vi "Actuate HW.vi"(8 "error in (no error)":errorcluster, 11 "DAQmx Servo in":refnum<class "DAQmx Servo.lvclass">) -> (0 "error out":errorcluster, 3 "DAQmx Servo out":refnum<class "DAQmx Servo.lvclass">)   [LabVIEW 2020, in "DAQmx Servo.lvclass"]
uses:
  DAQmx Servo.lvclass
  C:/Users/jharw/Documents/1 Folder to Rule them All/UMD/Inflation-Apparatus/src/Hardware/Actuators/Servos/Servo.lvclass
  Servo.lvclass/Servo.ctl
  DAQmx Servo.lvclass/DAQmx Servo.ctl
  <vilib>/DAQmx/write.llb/DAQmx Write (Counter Frequency 1Chan 1Samp).vi
  <vilib>/DAQmx/miscellaneous.llb/DAQmx Fill In Error Info.vi
  <resource>/objmgr/daqmx.rc
  Servo.lvclass
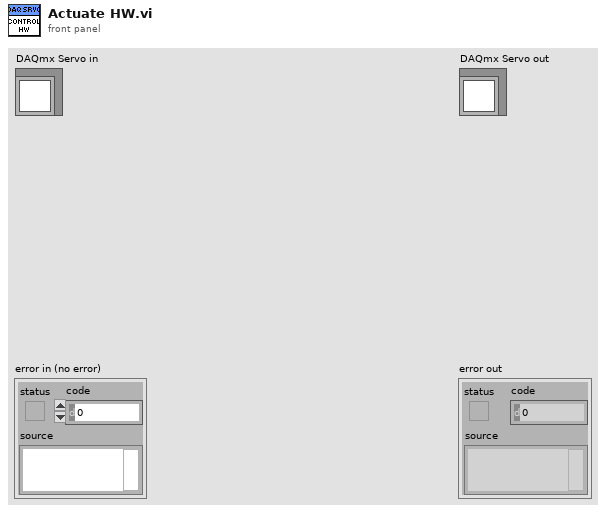
[diagram p1: front panel]
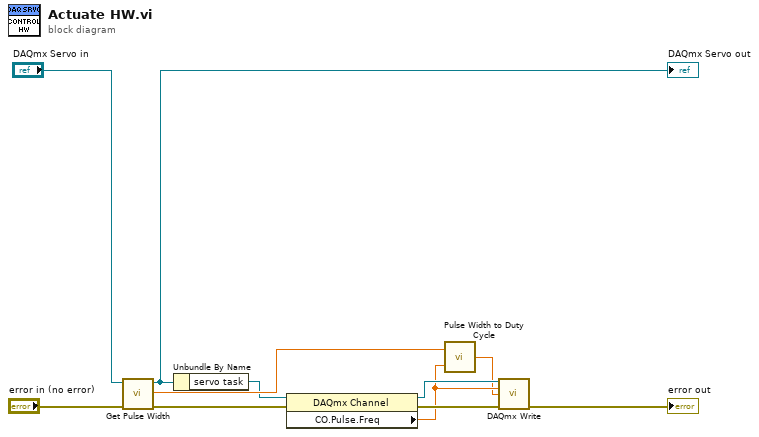
[diagram p0: block diagram]
diagram:
  n1 = call "Get Pulse Width.vi"("error in (no error)"="error in (no error)", "Servo in"="DAQmx Servo in") -> ("error out"=w7:errorcluster, "pulse width (micro-sec)"=w3:dbl, "Servo out"=w2:refnum<class "DAQmx Servo.lvclass">)  [unwired: 7 in]
  "DAQmx Servo out" <- w2
  n2 = Unbundle By Name(w2) -> ("servo task"=w1:refnum<k21>)
  n3 = property class="DAQmx Channel"(reference=w1, error in=w7) -> (reference out=w11:refnum<k21>, error out=w10:errorcluster, "CO.Pulse.Freq"=w9:dbl)
  n4 = call "Pulse Width to Duty Cycle.vi"("frequency"=w9, "pulse width (us)"=w3) -> ("duty cycle"=w8:dbl)
  n5 = call-poly <vilib>:"DAQmx Write.vi"("task/channels in"=w11, "frequency"=w9, "duty cycle"=w8, "error in"=w10) -> ("error out"=→"error out":errorcluster)  [unwired: 9 in, 2 out]
